vi "GET-HD-INFO.vi"() -> (3 "HDD SN":string, 4 "BIOS Info":string, 6 "BIOS SN":string, 8 "CPU SN":string, 10 "CPU Specification":string, 14 "MAC":string[](array[string]), 15 "CPU Manufacturers":string)   [LabVIEW 2014]
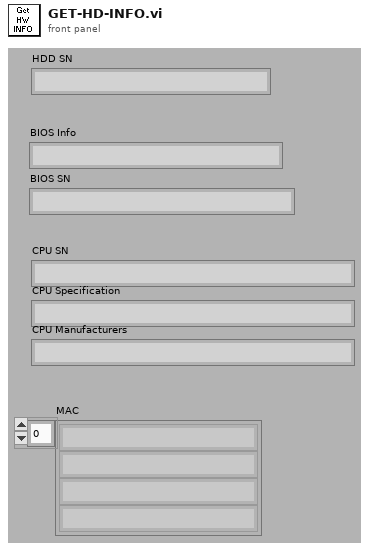
[diagram p1: front panel]
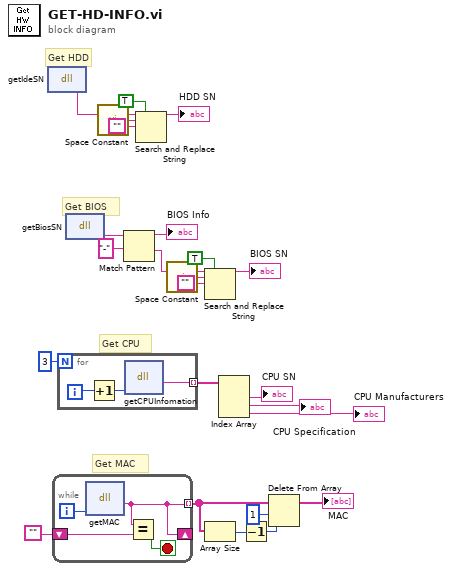
[diagram p0: block diagram]
diagram:
  # "Get MAC"
  # "Get CPU"
  # "Get BIOS"
  # "Get HDD"
  n1 = dll-call lib="PTH2Habs E项目本地部分模块化VI获取计算机SN\tGetHW.dll" fn="getIdeSN"() -> ("return type"=w24:string)  [unwired: 3 in, 2 out]
  n2 = while {
    shift-right: [w25] -> _
    shift-left: "" -> [w27]
    tunnel: [w25] -> w4 mode=indexing
    i -> [w28]
    stop <- w26 stop-if-true
    n3 = dll-call lib="PTH2Habs E项目本地部分模块化VI获取计算机SN\tGetHW.dll" fn="getMAC"("infoID"=w28) -> ("return type"=w25:string)  [unwired: 4 in, 2 out]
    n4 = Equal?(x=w25, y=w27) -> (x = y?=w26:bool)
  }
  n5 = for {
    N: 3 -> [_]
    tunnel: [w29] -> w10 mode=indexing
    i -> [w31]
    n6 = Increment(x=w31) -> (x+1=w30:i32)
    n7 = dll-call lib="PTH2Habs E项目本地部分模块化VI获取计算机SN\tGetHW.dll" fn="getCPUInfomation"("infoID"=w30) -> ("return type"=w29:string)  [unwired: 4 in, 2 out]
  }
  n8 = dll-call lib="PTH2Habs E项目本地部分模块化VI获取计算机SN\tGetHW.dll" fn="getBiosSN"() -> ("return type"=w19:string)  [unwired: 3 in, 2 out]
  n9 = call <vilib>:"Space Constant.vi"() -> ("String"=w22:string)
  n10 = Match Pattern(string=w19, regular expression="-") -> (before substring=→"BIOS Info":string, after substring=w14:string)  [unwired: 3 out]
  n11 = Search and Replace String(replace all?=TRUE ("replace all? (F)"), input string=w24, search string=w22, replace string="") -> (result string=→"HDD SN":string)  [unwired: 1 in, 6 out]
  n12 = call <vilib>:"Space Constant.vi"() -> ("String"=w16:string)
  n13 = Search and Replace String(replace all?=TRUE ("replace all? (F)"), input string=w14, search string=w16, replace string="") -> (result string=→"BIOS SN":string)  [unwired: 1 in, 6 out]
  n14 = Array Size(array=w4) -> (size(s)=w2:i32)
  n15 = Index Array(array=w10) -> (element #1=→"CPU SN":string, element #2=→"CPU Specification":string, element #3=→"CPU Manufacturers":string)  [unwired: 3 in]
  n16 = Decrement(x=w2) -> (x-1=w1:i32)
  n17 = Delete From Array(array=w4, length=1, index=w1) -> (array with subset deleted=→"MAC":string[])  [unwired: 1 out]
